vi "globalstop-example1.vi"() -> ()   [LabVIEW 2017]
uses:
  user.lib/_NEVSTOP/GlobalStop/_gStop.vi
  user.lib/_NEVSTOP/GlobalStop/GSTOP.lvlib
panel:
  in  "gen error":bool
  out "error out":errorcluster
  out "loop4":i32
  in  "stop 2":bool
  out "loop3":i32
  out "loop2":i32
  out "loop1":i32
  in  "stop":bool
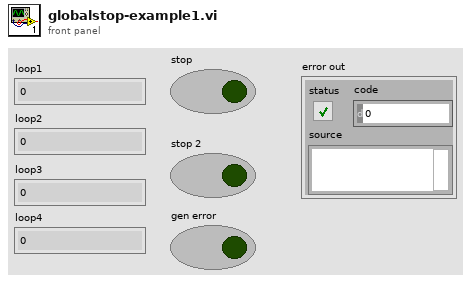
[diagram p1: front panel]
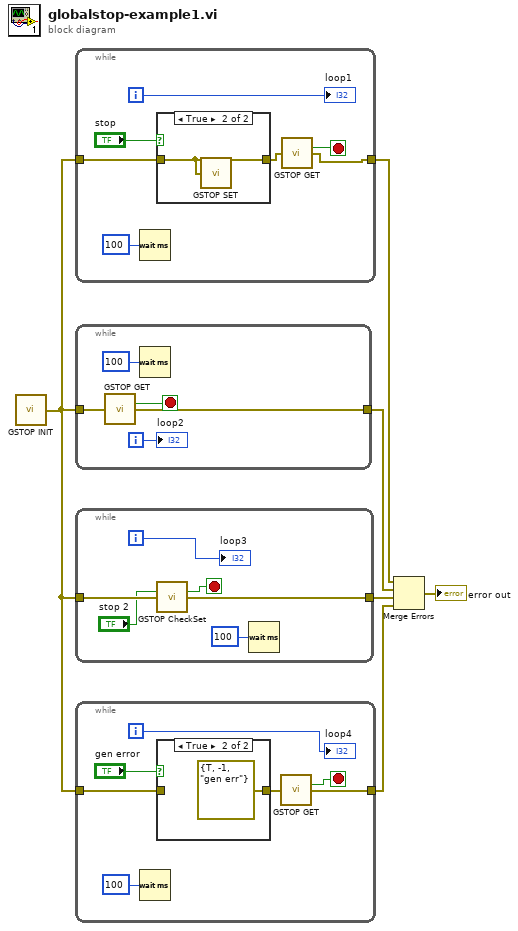
[diagram p0: block diagram]
diagram:
  n1 = call "GSTOP INIT.vi"() -> ("error out"=w3:errorcluster)  [unwired: 15 in]
  n2 = while {
    tunnel: w3 -> [w13]
    tunnel: [w8] -> w6
    i -> [w11]
    stop <- w7 stop-if-true
    n3 = Wait (ms)(milliseconds to wait=100) -> ()  [unwired: 1 out]
    n4 = case shown="True" "stop" {
      tunnel: w13 -> [w14 w15]
      tunnel: [w14 w15] -> w9
      frame False {
      }
      frame True {
        n5 = call "GSTOP SET.vi"("error in (no error)"=w15) -> ()  [unwired: 14 in, 1 out]
      }
    }
    n6 = call "GSTOP GET.vi"("error in (no error)"=w9) -> ("stop"=w7:bool, "error out"=w8:errorcluster)  [unwired: 13 in]
    "loop1" <- w11
  }
  n7 = while {
    tunnel: w3 -> [w18]
    tunnel: [w16] -> w5
    i -> [w20]
    stop <- w17 stop-if-true
    n8 = call "GSTOP GET.vi"("error in (no error)"=w18) -> ("stop"=w17:bool, "error out"=w16:errorcluster)  [unwired: 13 in]
    n9 = Wait (ms)(milliseconds to wait=100) -> ()  [unwired: 1 out]
    "loop2" <- w20
  }
  n10 = while {
    tunnel: w3 -> [w24]
    tunnel: [w23] -> w4
    i -> [w26]
    stop <- w22 stop-if-true
    n11 = call "GSTOP CheckSet.vi"("stop value"="stop 2", "error in (no error)"=w24) -> ("stop"=w22:bool, "error out"=w23:errorcluster)  [unwired: 12 in]
    n12 = Wait (ms)(milliseconds to wait=100) -> ()  [unwired: 1 out]
    "loop3" <- w26
  }
  n13 = while {
    tunnel: w3 -> [w30]
    tunnel: [w28] -> w2
    i -> [w33]
    stop <- w27 stop-if-true
    n14 = Wait (ms)(milliseconds to wait=100) -> ()  [unwired: 1 out]
    n15 = case shown="True" "gen error" {
      tunnel: w30 -> [w34 _]
      tunnel: [w34 errorcluster {"status"=TRUE, "code"=-1, "source"="gen err"} ("error out")] -> w29
      frame False {
      }
      frame True {
      }
    }
    n16 = call "GSTOP GET.vi"("error in (no error)"=w29) -> ("stop"=w27:bool, "error out"=w28:errorcluster)  [unwired: 13 in]
    "loop4" <- w33
  }
  n17 = Merge Errors(w6, w5, w4, w2) -> (→"error out":errorcluster)
